vi "Read DVM.vi"(8 "error in (no error)":errorcluster, 11 "Agilent 3054A in":refnum<class "Agilent 3054A.lvclass">) -> (0 "error out":errorcluster, 1 "5-digit Frequency":dbl, 2 "3-digit DVM":dbl, 3 "Agilent 3054A out":refnum<class "Agilent 3054A.lvclass">)   [LabVIEW 2021, in "Oscilloscope.lvlib" / "Agilent 3054A.lvclass"]
uses:
  Agilent 3054A.lvclass
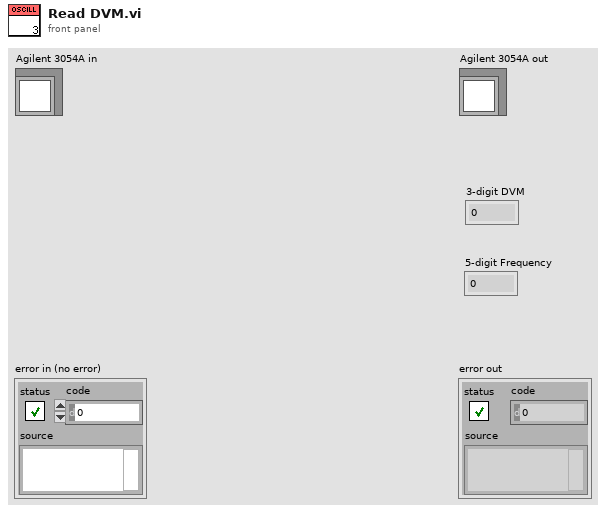
[diagram p1: front panel]
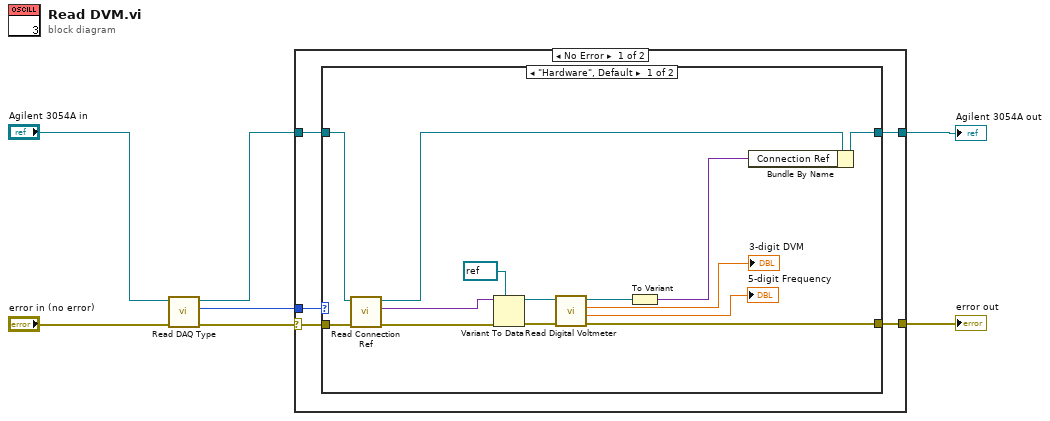
[diagram p0: block diagram]
diagram:
  n1 = call-dynamic "Read DAQ Type.vi"("error in (no error)"="error in (no error)", "Agilent 3054A in"="Agilent 3054A in") -> ("error out"=w6:errorcluster, "DAQ Type"=w4:enum16{"Hardware", "Simulation"}, "Agilent 3054A out"=w1:refnum<class "Agilent 3054A.lvclass">)  [unwired: 7 in]
  n2 = case shown="No Error" w6 {
    selector: w6 -> [w12 w29]
    tunnel: w1 -> [w10 w30]
    tunnel: w4 -> [w11 _]
    tunnel: [w9 w30] -> w2
    tunnel: [w8 w29] -> w3
    frame No Error {
      n3 = case shown="\"Hardware\", Default" w11 {
        tunnel: w12 -> [w26 w27]
        tunnel: w10 -> [w14 w28]
        tunnel: [w19 w28] -> w9
        tunnel: [w20 w27] -> w8
        frame "Hardware", Default {
          n4 = call-dynamic "Read Connection Ref.vi"("error in (no error)"=w26, "Agilent 3054A in"=w14) -> ("error out"=w25:errorcluster, "Connection Ref"=w24:variant, "Agilent 3054A out"=w13:refnum<class "Agilent 3054A.lvclass">)  [unwired: 7 in]
          n5 = Variant To Data(error in=w25, type=refnum<visa-resource-name> refnum ("VISA resource name"), Variant=w24) -> (data=w22:refnum<visa-resource-name>, error out=w21:errorcluster)
          n6 = call <instrlib>:"Read Digital Voltmeter.vi"("error in (no error)"=w21, "VISA resource name"=w22) -> ("error out"=w20:errorcluster, "5-digit Frequency"=→"5-digit Frequency":dbl, "3-digit DVM"=→"3-digit DVM":dbl, "VISA resource name out"=w18:refnum<visa-resource-name>)  [unwired: 6 in]
          n7 = To Variant(anything=w18) -> (Variant=w15:variant)
          n8 = Bundle By Name(cluster=w13, "Connection Ref"=w15) -> (w19:refnum<class "Agilent 3054A.lvclass">)
        }
        frame "Simulation" {
        }
      }
    }
    frame Error {
    }
  }
  "error out" <- w3
  "Agilent 3054A out" <- w2
